vi "Get Channels Timing.vi"(8 "error in (no error)":errorcluster, 11 "Data file":T2={"File path"=path "", "Channels"=[], "Group"="Untitled"}) -> (0 "error out":errorcluster, 2 "Channels info":T1[](array[typedef]), 4 "Latest finish":dbl, 5 "Plots exist":bool, 6 "Earliest start":dbl)   [LabVIEW 2016]
uses:
  Controls/Data Viewer Entry.ctl
  Controls/Channel name entry.ctl
  Controls/TDMS channel info.ctl
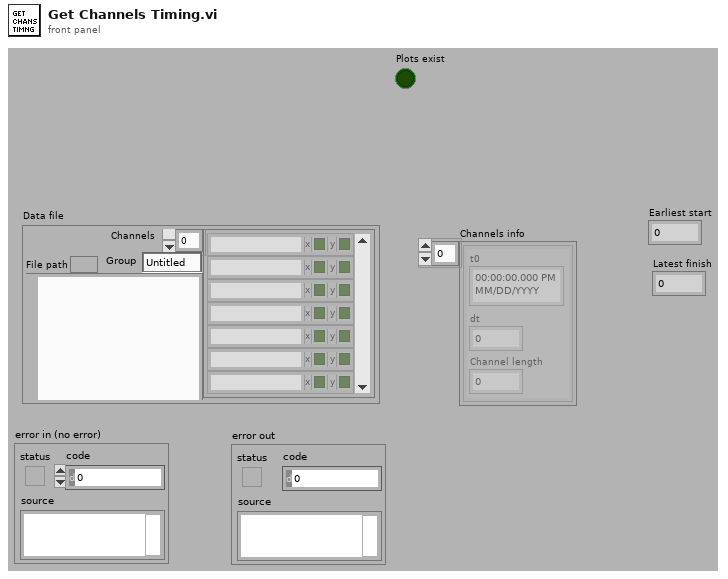
[diagram p1: front panel]
types:
  T1 = typedef "TDMS channel info.ctl" = cluster{"t0":timestamp, "dt":dbl, "Channel length":i64}
  T2 = typedef "Data Viewer Entry.ctl" = cluster{"File path":path, "Channels":T3[], "Group":string}
  T3 = typedef "Channel name entry.ctl" = cluster{"Name":string, "x":bool, "y":bool}
  T4 = enum16{"open", "open or create", "create or replace", "create", "open (read-only)"}
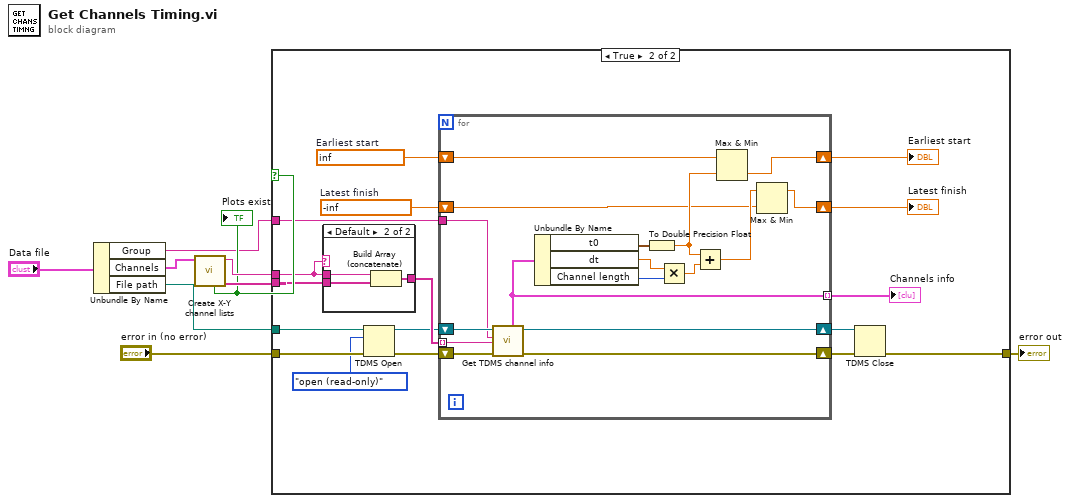
[diagram p0: block diagram]
diagram:
  n1 = Unbundle By Name("Data file") -> ("Group"=w1:string, "Channels"=w7:T3[], "File path"=w8:path)
  n2 = call "Create X-Y channel lists.vi"("Channels to plot"=w7) -> ("Y names"=w5:string[], "X-axis name"=w6:string, "Plots exist"=w2:bool)  [unwired: 6 in, 2 out]
  "Plots exist" <- w2
  n3 = case shown="True" w2 {
    tunnel: w8 -> [_ w27]
    tunnel: w6 -> [_ w13]
    tunnel: w5 -> [_ w25]
    tunnel: "error in (no error)" -> [w10 w15]
    tunnel: [w10 w14] -> w3
    tunnel: w1 -> [_ w11]
    frame False {
    }
    frame True {
      w20 = -inf  # Latest finish
      w21 = inf  # Earliest start
      n4 = case shown="Default" w13 {
        tunnel: w13 -> [_ w31]
        tunnel: w25 -> [w28 w30]
        tunnel: [w28 w29] -> w24
        frame "Time" {
        }
        frame Default {
          n5 = Build Array (concatenate)(w31, w30) -> (w29:string[])
        }
      }
      n6 = TDMS Open(8:w15, 10:T4."open (read-only)" ("operation (0:open)"), 11:w27) -> (0:w26:errorcluster, 3:w23:refnum<k34>)  [unwired: 4 in]
      n7 = for {
        tunnel: w24 -> [w47] mode=indexing
        shift-right: [w45] -> w17
        shift-left: w26 -> [w48]
        tunnel: [w43] -> w22 mode=indexing
        shift-right: [w40] -> w19
        shift-left: w21 -> [w41]
        shift-right: [w33] -> w18
        shift-left: w20 -> [w34]
        shift-right: [w44] -> w16
        shift-left: w23 -> [w46]
        tunnel: w11 -> [w32]
        n8 = call "Get TDMS channel info.vi"("error in"=w48, "Channel name"=w47, "group name"=w32, "tdms file"=w46) -> ("error out"=w45:errorcluster, "tdms file out"=w44:refnum<k34>, "TDMS channel info"=w43:T1)  [unwired: 3 in, 2 out]
        n9 = Unbundle By Name(w43) -> ("t0"=w42:timestamp, "dt"=w39:dbl, "Channel length"=w38:i64)
        n10 = To Double Precision Float(number=w42) -> (double precision float=w37:dbl)
        n11 = Multiply(x=w39, y=w38) -> (x*y=w36:dbl)
        n12 = Add(x=w37, y=w36) -> (x+y=w35:dbl)
        n13 = Max & Min(x=w41, y=w37) -> (min(x,y)=w40:dbl)  [unwired: 1 out]
        n14 = Max & Min(x=w35, y=w34) -> (max(x,y)=w33:dbl)  [unwired: 1 out]
      }
      "Channels info" <- w22
      "Earliest start" <- w19
      "Latest finish" <- w18
      n15 = TDMS Close(8:w17, 11:w16) -> (0:w14:errorcluster)  [unwired: 1 out]
    }
  }
  "error out" <- w3
